vi "Get All Items.vi"(8 "error in (no error)":errorcluster, 11 "JSON Value In":refnum<class "JSON Value.lvclass">) -> (0 "error out":errorcluster, 1 "Values":refnum<class "JSON Value.lvclass">[](array[class]), 2 "Item Names":string[](array[string]), 3 "JSON Value Out":refnum<class "JSON Value.lvclass">)   [LabVIEW 2020, in "Library Commun.lvlib" / "JSON Value.lvclass"]
doc: "Returns the names of the Object's elements.\n\nCopyright 2012 James David Powell, Shaun Rumbell and Ton Plomp\nMore information on http://lavag.org/topic/16217-cr-json-labview"
uses:
  JSON Value.lvclass
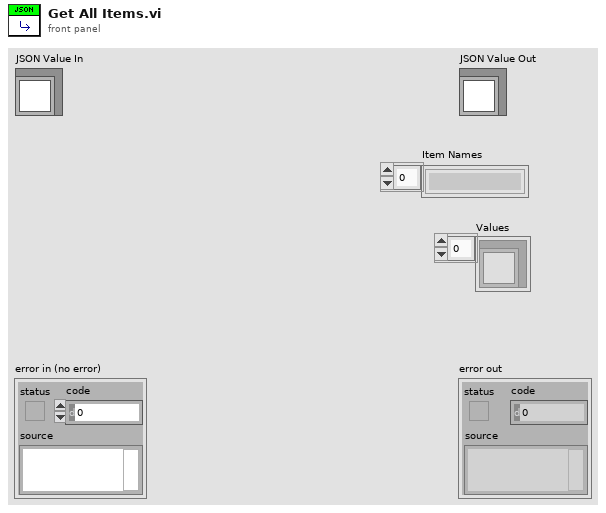
[diagram p1: front panel]
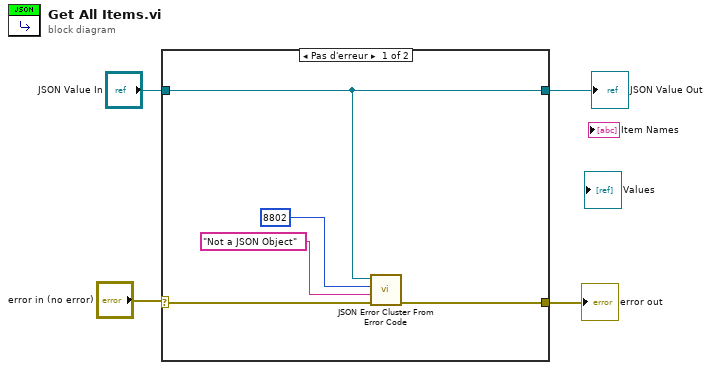
[diagram p0: block diagram]
diagram:
  n1 = case shown="Pas d'erreur" "error in (no error)" {
    selector: "error in (no error)" -> [w7 w11]
    tunnel: [w8 w11] -> w1
    tunnel: [w9 w10] -> w3
    tunnel: "JSON Value In" -> [w9 w10]
    frame No Error {
      n2 = call "JSON Error Cluster From Error Code.vi"("error in (no error)"=w7, "Error message"="Not a JSON Object", "JSON error code"=8802, "JSON Value in"=w9) -> ("error out"=w8:errorcluster)  [unwired: 6 in, 1 out]
    }
    frame Error {
    }
  }
  "error out" <- w1
  "JSON Value Out" <- w3
